vi "get live autosave boolean from DB.vi"(11 ">Expt Name >":string) -> (3 "save live config":bool)   [LabVIEW 2020]
panel:
  out "concatenated string":string
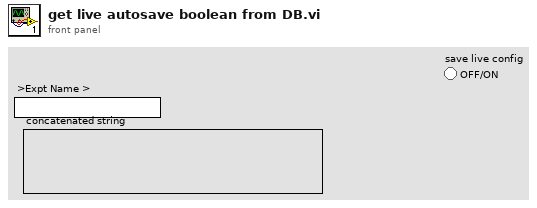
[diagram p1: front panel]
types:
  T1 = typedef "mysql_authentication.ctl" = cluster{"User":string, "Password":string, "Database":string}
  T2 = cluster{"Port":u16, "IP Address":string, "Authentication":T1}
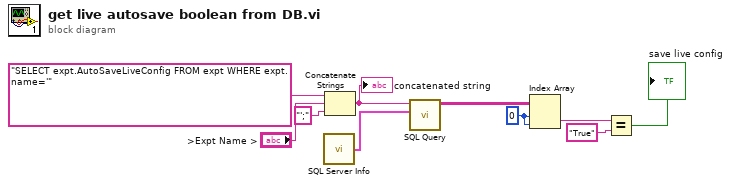
[diagram p0: block diagram]
diagram:
  w7 = 0
  n1 = call "SQL Server Info.vi"() -> ("SQL Server Info"=w1:T2)
  n2 = Concatenate Strings("SELECT expt.AutoSaveLiveConfig FROM expt WHERE expt.name='" ("Query"), ">Expt Name >", "';" ("element")) -> (w5:string)
  "concatenated string" <- w5
  n3 = call "SQL Query.vi"("SQL Server Info"=w1, "Query"=w5) -> ("data"=w6:string[][])  [unwired: 8 in, 1 out]
  n4 = Index Array(array=w6, index (row)=w7, index (col)=w7) -> (element=w8:string)
  n5 = Equal?(x=w8, y="True") -> (x = y?=→"save live config":bool)
